vi "Simple Motor Feedforward.vi"(8 "Reset? (F)":bool, 9 "dt":dbl, 10 "Feed Forward Constants":cluster{"kS":dbl, "kV":dbl, "kA":dbl}, 11 "Velocity Reference":dbl format="%#_13g") -> (3 "Feedforward":dbl)   [LabVIEW 2019]
panel:
  in  "Reset? (F)":bool
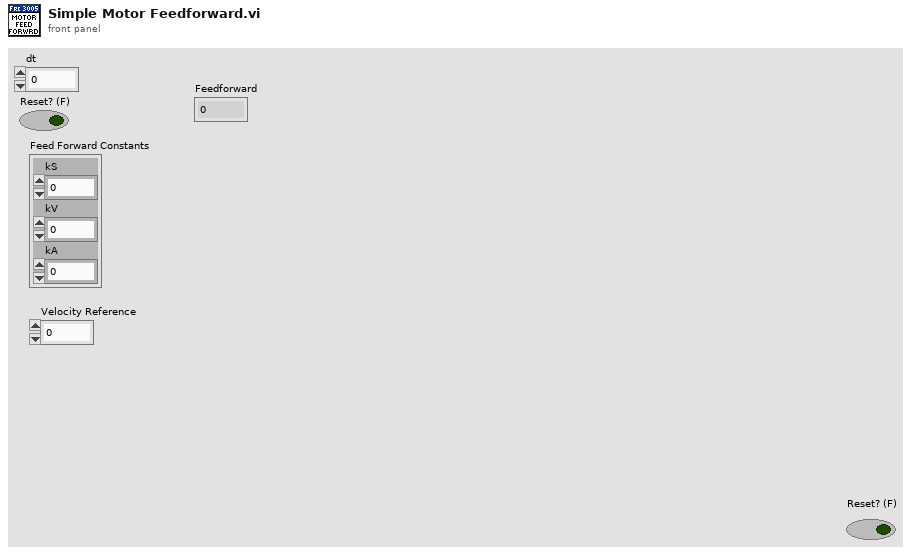
[diagram p1: front panel]
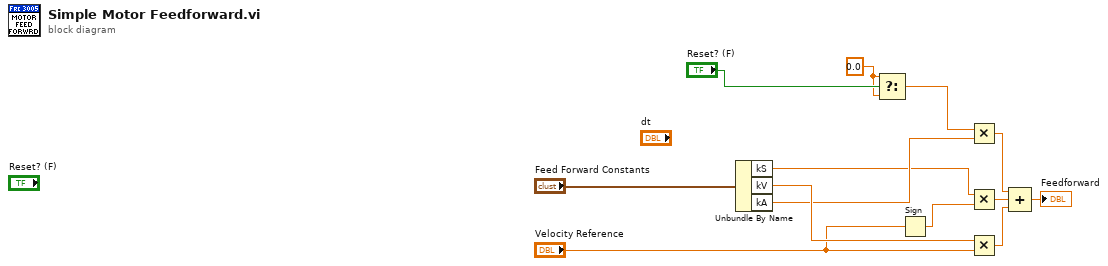
[diagram p0: block diagram]
diagram:
  w1 = 0.0 ("t")
  n1 = Unbundle By Name("Feed Forward Constants") -> ("kS"=w4:dbl, "kV"=w11:dbl, "kA"=w10:dbl)
  n2 = Select(t=w1, s="Reset? (F)", f=w1) -> (s? t:f=w5:dbl)
  n3 = Sign(1:"Velocity Reference") -> (0:w12:dbl)
  n4 = Multiply(x=w5, y=w10) -> (x*y=w9:dbl)
  n5 = Multiply(x=w4, y=w12) -> (x*y=w7:dbl)
  n6 = Multiply(x=w11, y="Velocity Reference") -> (x*y=w8:dbl)
  n7 = Compound Arithmetic op=ADD(w9, w7, w8) -> (→"Feedforward":dbl)
